vi "wip2.vi"() -> ()   [LabVIEW 2021]
uses:
  <vilib>/Analysis/Matrix/Datatypes/RealMatrix.ctl
  <vilib>/Analysis/baseanly.llb/Real A x B.vi
  <vilib>/Analysis/NI_AALBase.lvlib
  <vilib>/Analysis/Matrix/NI_Matrix.lvlib
panel:
  out "Observation":dbl[][](array[numeric])=[[1.0], [0.0]]
  out "A x B":T1
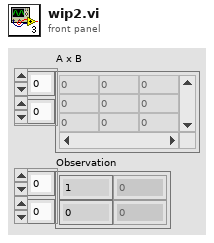
[diagram p1: front panel]
types:
  T1 = typedef "NI_Matrix.lvlib/RealMatrix.ctl" = dbl[][]
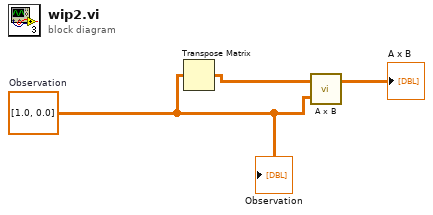
[diagram p0: block diagram]
diagram:
  w3 = dbl[][] [[1.0], [0.0]]  # Observation
  n1 = Transpose Matrix(1:w3) -> (0:w2:dbl[][])
  n2 = call-poly <vilib>:"A x B.vi"("B"=w3, "A"=w2) -> ("A x B"=→"A x B":T1)  [unwired: 1 out]
  "Observation" <- w3
